vi "WSVCAP SHL Host LL SPI Write_Read - Multiple DUTs - Common Data.vi"(0 "Data Out [U16]":u16 format="%04x", 11 "error in":errorcluster, 13 "DUT Mask (All)":bool[](array[boolean])=[TRUE, TRUE, TRUE, TRUE, TRUE, TRUE, TRUE, TRUE, TRUE, TRUE, TRUE, TRUE, TRUE, TRUE, TRUE, TRUE]) -> (4 "SPI Data In [U16]":u16[](array[numeric]) format="%04x", 15 "error out":errorcluster)   [LabVIEW 2012]
panel:
  out "SPI Data In [U8]":u8[][](array[numeric]) format="%02x"
  out "Socket Mask":u16=1 format="%02x"
  out "SPI Data Out [U8]":u8[][](array[numeric]) format="%02x"
  # "DUT 01"
  # "DUT 02"
  # "DUT 03"
  # "DUT 04"
  # "DUT 05"
  # "DUT 06"
  # "DUT 07"
  # "DUT 08"
  # "DUT 09"
  # "DUT 10"
  # "DUT 11"
  # "DUT 12"
  # "DUT 13"
  # "DUT 14"
  # "DUT 15"
  # "DUT 16"
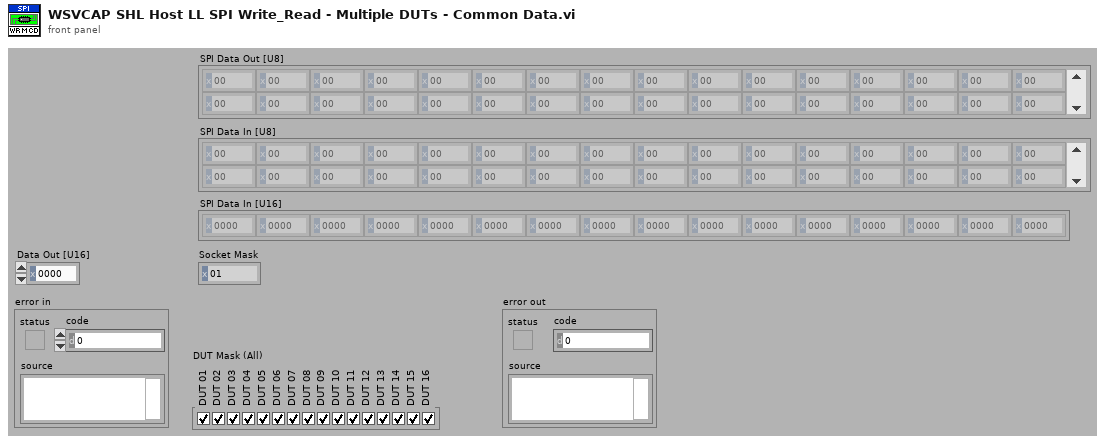
[diagram p1: front panel]
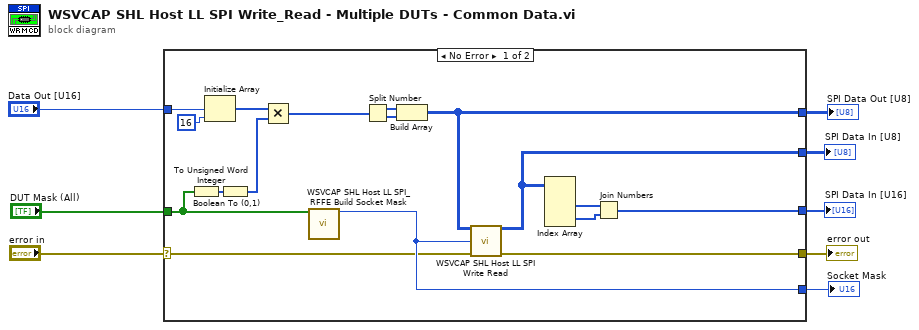
[diagram p0: block diagram]
diagram:
  n1 = case shown="No Error" "error in" {
    selector: "error in" -> [w9 _]
    tunnel: [w25 _] -> w8
    tunnel: "Data Out [U16]" -> [w17 _]
    tunnel: [w23 _] -> w5
    tunnel: [w24 _] -> w4
    tunnel: "DUT Mask (All)" -> [w14 _]
    tunnel: [w21 _] -> w2
    tunnel: [w18 _] -> w1
    frame No Error {
      n2 = Boolean To (0,1)(Boolean=w14) -> (0, 1=w13:i16[])
      n3 = Initialize Array(w17, 16 ("dimension size")) -> (w11:u16[])
      n4 = To Unsigned Word Integer(number=w13) -> (unsigned 16bit integer=w12:u16[])
      n5 = Multiply(x=w11, y=w12) -> (x*y=w10:u16[])
      n6 = call "WSVCAP SHL Host LL SPI_RFFE Build Socket Mask.vi"("DUT Mask"=w14) -> ("Socket Mask [U16]"=w24:u16)  [unwired: 13 in, 1 out]
      n7 = Split Number(x=w10) -> (hi(x)=w16:u8[], lo(x)=w15:u8[])
      n8 = Build Array(w16, w15) -> (w23:u8[][])
      n9 = call "WSVCAP SHL Host LL SPI Write Read.vi"("SPI Data [DUT Ordered]"=w23, "Cycle CMD Lengths Out (bits)"=w24, "error in"=w9) -> ("SPI Read Data [DUT Ordered]"=w21:u8[][], "error out"=w25:errorcluster)  [unwired: 10 in, 1 out]
      n10 = Index Array(array=w21) -> (element #1=w20:u8[], element #2=w19:u8[])  [unwired: 4 in]
      n11 = Join Numbers(hi=w20, lo=w19) -> ((hi.lo)=w18:u16[])
    }
    frame Error {
    }
  }
  "error out" <- w8
  "SPI Data Out [U8]" <- w5
  "Socket Mask" <- w4
  "SPI Data In [U16]" <- w1
  "SPI Data In [U8]" <- w2
